vi "Automatic CE-CERT Inverter MODBUS TCP-IP Curtailment.vi"() -> ()   [LabVIEW 2018]
uses:
  <vilib>/Plasmionique/MB Master/MB_Master_TCP/MB_Master_TCP.lvclass
  C:/Program Files (x86)/National Instruments/LabVIEW 2018/vi.lib/Plasmionique/MB Master/MB_Master/MB_Master.lvclass
  <vilib>/Plasmionique/MB Master/MB Master.lvlib
panel:
  in  "Seconds to wait between sent commands":u32
  in  "Number of Iterations":i32
  in  "Curtailment Percentage (28-100%)":u16
  out "3035 Register Value":u16
  out "Curtailment Mode Read Back (Step 11)":u16
  out "Power Factor Mode Read Back (Step 10)":u16
  out "Power Factor Operation Error (Step 9)(Can Read 0 or 10)":u16
  out "Power Factor Operation Error (Step 1)(Should Read 0)":u16
  in  "IP Address":string
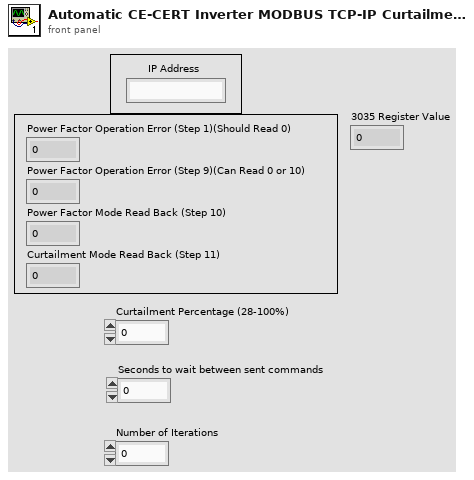
[diagram p1: front panel]
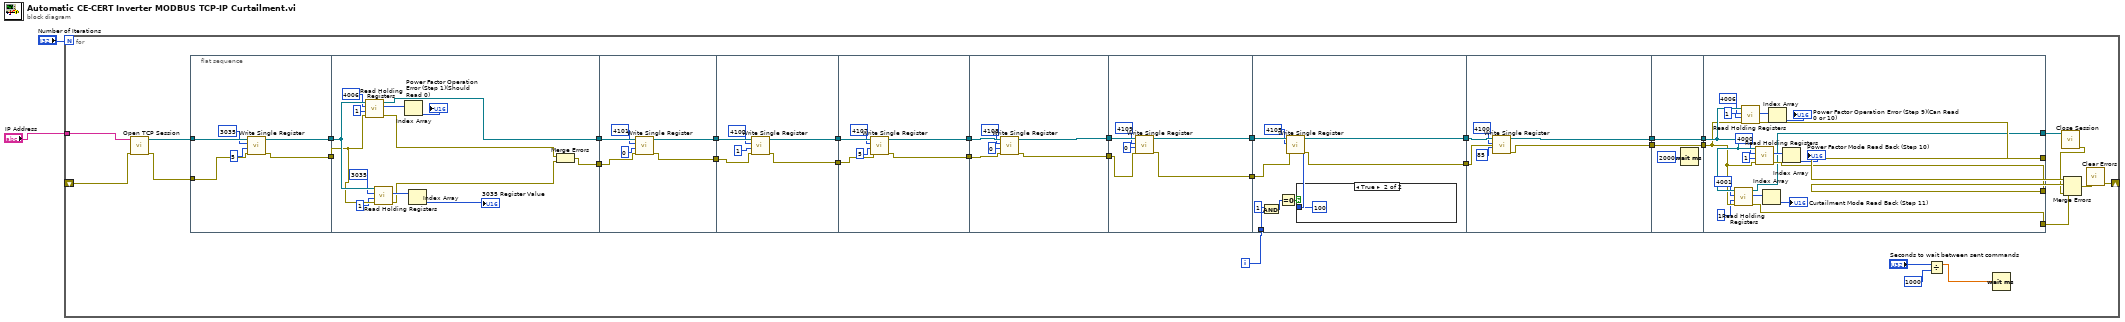
[diagram p0: block diagram]
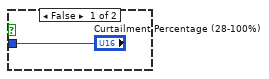
[diagram p2: hidden frame]
diagram:
  n1 = for {
    N: "Number of Iterations" -> [_]
    tunnel: "IP Address" -> [w35]
    shift-right: [w27] -> _
    shift-left: _ -> [w26]
    i -> [w6]
    n2 = call <vilib>:"Open TCP Session.vi"("error in (no error)"=w26, "IP Address"=w35) -> ("error out"=w33:errorcluster, "MB_TCP session"=w34:refnum<class "MB_Master_TCP.lvclass">)  [unwired: 8 in]
    n3 = flat-sequence {
      tunnel: w34 -> [w43]
      tunnel: [w42] -> w25
      tunnel: w33 -> [w41]
      tunnel: [w40] -> w24
      tunnel: [w57] -> w23
      tunnel: w25 -> [w56]
      tunnel: w24 -> [w55]
      tunnel: [w46] -> w22
      tunnel: w23 -> [w63]
      tunnel: [w62] -> w21
      tunnel: w22 -> [w61]
      tunnel: [w60] -> w20
      tunnel: w21 -> [w69]
      tunnel: [w68] -> w19
      tunnel: w20 -> [w67]
      tunnel: [w66] -> w18
      tunnel: w19 -> [w75]
      tunnel: [w74] -> w17
      tunnel: w18 -> [w73]
      tunnel: [w72] -> w16
      tunnel: w17 -> [w81]
      tunnel: [w80] -> w15
      tunnel: w16 -> [w79]
      tunnel: [w78] -> w14
      tunnel: w15 -> [w87]
      tunnel: [w86] -> w13
      tunnel: w14 -> [w85]
      tunnel: [w84] -> w12
      tunnel: w13 -> [w97]
      tunnel: [w96] -> w11
      tunnel: w12 -> [w95]
      tunnel: [w94] -> w10
      tunnel: w6 -> [w91]
      tunnel: w11 -> [w105]
      tunnel: [w104] -> w37
      tunnel: w10 -> [w103]
      tunnel: [w102] -> w31
      tunnel: w37 -> [w108]
      tunnel: [w108] -> w36
      tunnel: [w106] -> w32
      tunnel: w31 -> [w106]
      tunnel: w36 -> [w126]
      tunnel: w32 -> [w125]
      tunnel: [w124] -> w30
      tunnel: [w123] -> w29
      tunnel: [w122] -> w28
      tunnel: [w109] -> w3
      frame #0 {
        n4 = call <vilib>:"Write Single Register.vi"("error in (no error)"=w41, "value"=u16 5, "address"=u16 3035, "MB session in"=w43) -> ("error out"=w40:errorcluster, "MB session out"=w42:refnum<class "MB_Master_TCP.lvclass">)  [unwired: 6 in]
      }
      frame #1 {
        n5 = call <vilib>:"Read Holding Registers.vi"("error in (no error)"=w55, "quantity"=u16 1, "starting address"=u16 4006, "MB session in"=w56) -> ("error out"=w45:errorcluster, "Registers"=w50:u16[], "MB session out"=w57:refnum<class "MB_Master_TCP.lvclass">)  [unwired: 5 in]
        n6 = call <vilib>:"Read Holding Registers.vi"("error in (no error)"=w55, "quantity"=u16 1, "starting address"=u16 3035, "MB session in"=w56) -> ("error out"=w44:errorcluster, "Registers"=w52:u16[])  [unwired: 5 in, 1 out]
        n7 = Index Array(array=w50) -> (element=→"Power Factor Operation Error (Step 1)(Should Read 0)":u16)  [unwired: 1 in]
        n8 = Index Array(array=w52) -> (element=→"3035 Register Value":u16)  [unwired: 1 in]
        n9 = Merge Errors(w45, w44) -> (w46:errorcluster)
      }
      frame #2 {
        n10 = call <vilib>:"Write Single Register.vi"("error in (no error)"=w61, "value"=u16 0, "address"=u16 4101, "MB session in"=w63) -> ("error out"=w60:errorcluster, "MB session out"=w62:refnum<class "MB_Master_TCP.lvclass">)  [unwired: 6 in]
      }
      frame #3 {
        n11 = call <vilib>:"Write Single Register.vi"("error in (no error)"=w67, "value"=u16 1, "address"=u16 4102, "MB session in"=w69) -> ("error out"=w66:errorcluster, "MB session out"=w68:refnum<class "MB_Master_TCP.lvclass">)  [unwired: 6 in]
      }
      frame #4 {
        n12 = call <vilib>:"Write Single Register.vi"("error in (no error)"=w73, "value"=u16 5, "address"=u16 4107, "MB session in"=w75) -> ("error out"=w72:errorcluster, "MB session out"=w74:refnum<class "MB_Master_TCP.lvclass">)  [unwired: 6 in]
      }
      frame #5 {
        n13 = call <vilib>:"Write Single Register.vi"("error in (no error)"=w79, "value"=u16 0, "address"=u16 4108, "MB session in"=w81) -> ("error out"=w78:errorcluster, "MB session out"=w80:refnum<class "MB_Master_TCP.lvclass">)  [unwired: 6 in]
      }
      frame #6 {
        n14 = call <vilib>:"Write Single Register.vi"("error in (no error)"=w85, "value"=u16 0, "address"=u16 4109, "MB session in"=w87) -> ("error out"=w84:errorcluster, "MB session out"=w86:refnum<class "MB_Master_TCP.lvclass">)  [unwired: 6 in]
      }
      frame #7 {
        n15 = And(x=1, y=w91) -> (x .and. y?=w89:i32)
        n16 = Equal To 0?(x=w89) -> (x = 0?=w88:bool)
        n17 = case shown="True" w88 {
          tunnel: ["Curtailment Percentage (28-100%)" u16 100 ("Curtailment Percentage (28-100%)")] -> w92
          frame False {
          }
          frame True {
          }
        }
        n18 = call <vilib>:"Write Single Register.vi"("error in (no error)"=w95, "value"=w92, "address"=u16 4105, "MB session in"=w97) -> ("error out"=w94:errorcluster, "MB session out"=w96:refnum<class "MB_Master_TCP.lvclass">)  [unwired: 6 in]
      }
      frame #8 {
        n19 = call <vilib>:"Write Single Register.vi"("error in (no error)"=w103, "value"=u16 85, "address"=u16 4100, "MB session in"=w105) -> ("error out"=w102:errorcluster, "MB session out"=w104:refnum<class "MB_Master_TCP.lvclass">)  [unwired: 6 in]
      }
      frame #9 {
        n20 = Wait (ms)(milliseconds to wait=u32 2000) -> ()  [unwired: 1 out]
      }
      frame #10 {
        n21 = call <vilib>:"Read Holding Registers.vi"("error in (no error)"=w125, "quantity"=u16 1, "starting address"=u16 4001, "MB session in"=w126) -> ("error out"=w122:errorcluster, "Registers"=w111:u16[], "MB session out"=w109:refnum<class "MB_Master_TCP.lvclass">)  [unwired: 5 in]
        n22 = call <vilib>:"Read Holding Registers.vi"("error in (no error)"=w125, "quantity"=u16 1, "starting address"=u16 4006, "MB session in"=w126) -> ("error out"=w124:errorcluster, "Registers"=w119:u16[])  [unwired: 5 in, 1 out]
        n23 = call <vilib>:"Read Holding Registers.vi"("error in (no error)"=w125, "quantity"=u16 1, "starting address"=u16 4000, "MB session in"=w126) -> ("error out"=w123:errorcluster, "Registers"=w115:u16[])  [unwired: 5 in, 1 out]
        n24 = Index Array(array=w111) -> (element=→"Curtailment Mode Read Back (Step 11)":u16)  [unwired: 1 in]
        n25 = Index Array(array=w119) -> (element=→"Power Factor Operation Error (Step 9)(Can Read 0 or 10)":u16)  [unwired: 1 in]
        n26 = Index Array(array=w115) -> (element=→"Power Factor Mode Read Back (Step 10)":u16)  [unwired: 1 in]
      }
    }
    n27 = Divide(x="Seconds to wait between sent commands", y=u32 1000) -> (x/y=w8:dbl)
    n28 = Wait (ms)(milliseconds to wait=w8) -> ()  [unwired: 1 out]
    n29 = call-dynamic "Close Session.vi"("MB TCP session"=w3) -> ("error out"=w4:errorcluster)  [unwired: 10 in]
    n30 = Merge Errors(w30, w29, w28, w4) -> (w5:errorcluster)
    n31 = call <vilib>:"Clear Errors.vi"("error in (no error)"=w5) -> ("error out"=w27:errorcluster)  [unwired: 5 in, 1 out]
  }
